vi "ServiceOrderQRcode (Get).vi"(7 "LabVIEW Web Service Request":refnum<class "Web Request.lvclass">) -> ()   [LabVIEW 2019]
uses:
  <vilib>/wsapi/Web Request.lvclass
  QDMH support files/QDMH Poly VIs/QDMH POLY Enqueue String.vi
panel:
  # "Use the Web Service Request input terminal to call the VIs on the Web Services palette. Do not remove it from the connector pane unless you don't need access to the palette."
  # "Each additional control wired to the connector pane will be available as an input in the URL. To include an indicator in terminal-mode output (the default setting), it must also be wired to the connector pane."
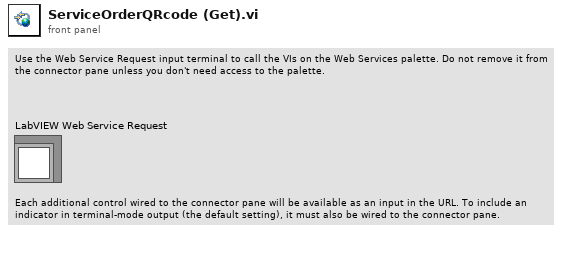
[diagram p1: front panel]
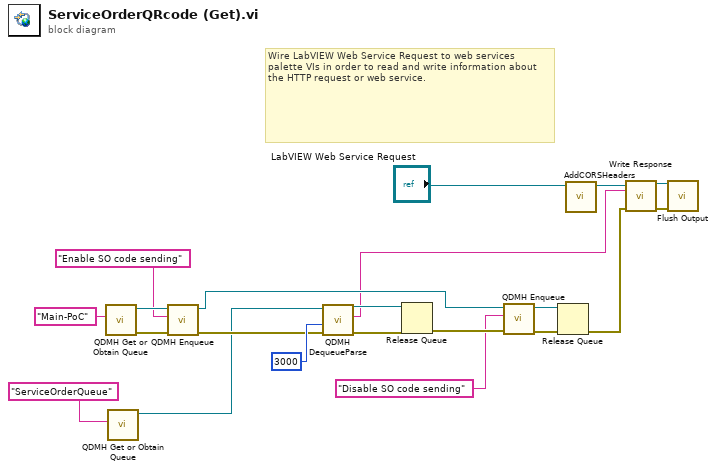
[diagram p0: block diagram]
diagram:
  # "Wire LabVIEW Web Service Request to web services palette VIs in order to read and write information about the HTTP request or web service."
  n1 = call "QDMH Get or Obtain Queue.vi"("Queue Name"="Main-PoC") -> ("error out"=w15:errorcluster, "queue out"=w16:refnum<queue>)  [unwired: 2 in, 7 out]
  n2 = call "QDMH Get or Obtain Queue.vi"("Queue Name"="ServiceOrderQueue") -> ("queue out"=w8:refnum<queue>)  [unwired: 2 in, 8 out]
  n3 = call-poly "QDMH Enqueue.vi"("error in (no error)"=w15, "State"="Enable SO code sending", "queue"=w16) -> ("error out"=w9:errorcluster, "queue out"=w6:refnum<queue>)  [unwired: 7 out]
  n4 = call "QDMH DequeueParse.vi"("error in (no error)"=w9, "Timeout"=3000, "queue"=w8) -> ("error out"=w11:errorcluster, "State"=w4:string, "queue out"=w10:refnum<queue>)  [unwired: 5 in, 1 out]
  n5 = Release Queue(queue=w10, error in (no error)=w11) -> (error out=w7:errorcluster)  [unwired: 1 in, 2 out]
  n6 = call-poly "QDMH Enqueue.vi"("error in (no error)"=w7, "State"="Disable SO code sending", "queue"=w6) -> ("error out"=w3:errorcluster, "queue out"=w1:refnum<queue>)  [unwired: 7 out]
  n7 = Release Queue(queue=w1, error in (no error)=w3) -> (error out=w2:errorcluster)  [unwired: 1 in, 2 out]
  n8 = call "AddCORSHeaders.vi"("Web Request in"="LabVIEW Web Service Request") -> ("Web Request out"=w19:refnum<class "Web Request.lvclass">)  [unwired: 10 in]
  n9 = call <vilib>:"Write Response.vi"("LabVIEW Web Service Request"=w19, "response string"=w4, "error in (no error)"=w2) -> ("LabVIEW Web Service Request out"=w21:refnum<class "Web Request.lvclass">, "error out"=w20:errorcluster)  [unwired: 11 in]
  n10 = call <vilib>:"Flush Output.vi"("LabVIEW Web Service Request"=w21, "error in (no error)"=w20) -> ()  [unwired: 12 in, 2 out]
